vi "niScope Adjust Sample Clock Relative Delay.vi"(0 "instrument handle":refnum<k15>, 5 "delay":dbl format="%^.4e", 11 "error in":errorcluster) -> (4 "instrument handle out":refnum<k15>, 15 "error out":errorcluster)   [LabVIEW 2011]
doc: "Configures the relative sample clock delay (in seconds) when using the internal clock. Each time this VI is called, the Sample Clock is delayed from the Reference clock by the specified amount of time."
uses:
  niScope_32.dll
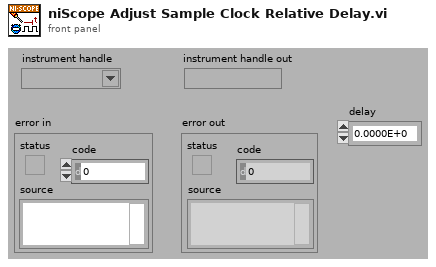
[diagram p1: front panel]
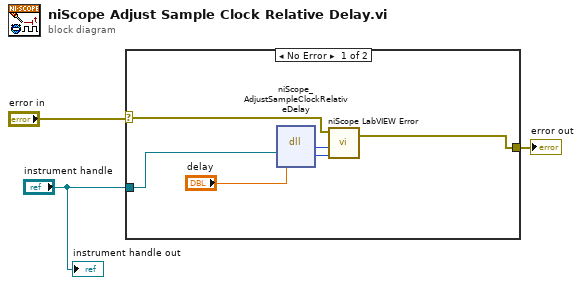
[diagram p0: block diagram]
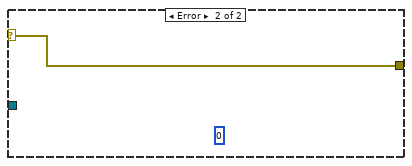
[diagram p2: hidden frame]
diagram:
  n1 = case shown="No Error" "error in" {
    selector: "error in" -> [w5 w10]
    tunnel: [w6 w10] -> w3
    tunnel: "instrument handle" -> [w9 _]
    frame No Error {
      n2 = dll-call lib="niScope_*.*" fn="niScope_AdjustSampleClockRelativeDelay"("instrument handle"=w9, "delay"="delay") -> ("status"=w7:i32, "instrument handle"=w8:u32)  [unwired: 4 in, 2 out]
      n3 = call <instrlib>:"niScope LabVIEW Error.vi"("instrument handle"=w8, "niScope error code (0)"=w7, "error in (no error)"=w5) -> ("error out"=w6:errorcluster)  [unwired: 2 in]
    }
    frame Error {
      (unwired) 0 ("actual  record length")
    }
  }
  "error out" <- w3
  "instrument handle out" <- "instrument handle"
